vi "Parse Fix Type.vi"(10 "Fix Index":i32, 11 "Fields In":string[](array[string])) -> (2 "Fix Type":T1, 3 "Fields":string[](array[string]))   [LabVIEW 2020, in "nmea.lvlib" / "nmea.lvclass"]
uses:
  nmea.lvclass
  Fix Type.ctl
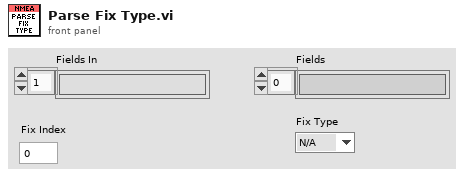
[diagram p1: front panel]
types:
  T1 = typedef "nmea.lvlib/nmea.lvclass/Fix Type.ctl" = enum16{"N/A", "None", "2D", "3D"}
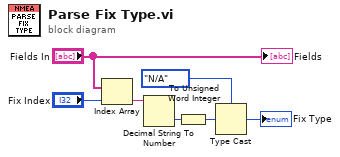
[diagram p0: block diagram]
diagram:
  n1 = Index Array(array="Fields In", index="Fix Index") -> (element=w5:string)
  n2 = Decimal String To Number(string=w5) -> (number=w4:i32)  [unwired: 2 in, 1 out]
  n3 = To Unsigned Word Integer(number=w4) -> (unsigned 16bit integer=w1:u16)
  n4 = Type Cast(type=Fix_Type."N/A" ("Fix Type"), x=w1) -> (*(type *) &x=→"Fix Type":T1)
  "Fields" <- "Fields In"
